vi "send_message_SIM921.vi"(8 "error in (no error)":errorcluster, 9 "Message (\"\")":string="\"\"", 10 "Channel (0: SIM900)":i32(ring) items=["SIM900", "1", "2", "3", "4", "5", "6", "7", "8", "9", "A", "B", "C", "D"], 11 "VISA resource name":refnum<visa-resource-name>) -> (0 "error out":errorcluster, 3 "VISA resource name out":refnum<visa-resource-name>)   [LabVIEW 2019]
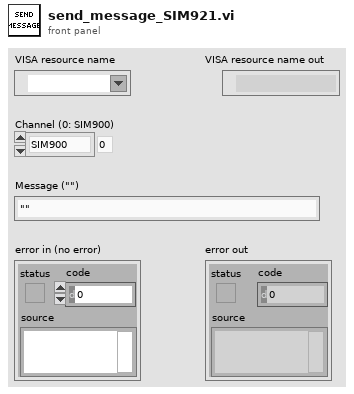
[diagram p1: front panel]
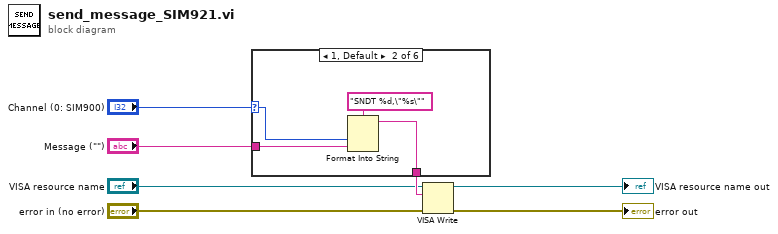
[diagram p0: block diagram]
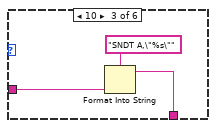
[diagram p3: hidden frame]
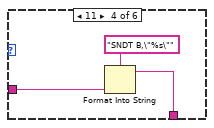
[diagram p4: hidden frame]
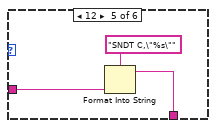
[diagram p5: hidden frame]
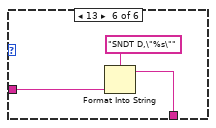
[diagram p6: hidden frame]
diagram:
  n1 = case shown="1, Default" "Channel (0: SIM900)" {
    selector: "Channel (0: SIM900)" -> [_ w9 _ _ _ _]
    tunnel: "Message (\"\")" -> [w8 w11 w13 w16 w19 w22]
    tunnel: [w8 w10 w14 w17 w20 w23] -> w6
    frame 0 {
    }
    frame 1, Default {
      n2 = Format Into String(format string="SNDT %d,\"%s\"", w9, w11) -> (resulting string=w10:string)  [unwired: 2 in, 1 out]
    }
    frame 10 {
      n3 = Format Into String(format string="SNDT A,\"%s\"", w13) -> (resulting string=w14:string)  [unwired: 2 in, 1 out]
    }
    frame 11 {
      n4 = Format Into String(format string="SNDT B,\"%s\"", w16) -> (resulting string=w17:string)  [unwired: 2 in, 1 out]
    }
    frame 12 {
      n5 = Format Into String(format string="SNDT C,\"%s\"", w19) -> (resulting string=w20:string)  [unwired: 2 in, 1 out]
    }
    frame 13 {
      n6 = Format Into String(format string="SNDT D,\"%s\"", w22) -> (resulting string=w23:string)  [unwired: 2 in, 1 out]
    }
  }
  n7 = VISA Write(VISA resource name="VISA resource name", write buffer=w6, error in (no error)="error in (no error)") -> (VISA resource name out=→"VISA resource name out":refnum<visa-resource-name>, error out=→"error out":errorcluster)  [unwired: 1 out]
